vi "Configure Math.vi"(0 "VISA resource name":refnum<visa-resource-name>, 1 "Operation (0:None)":T1(ring), 2 "Internal Math Buffer Storage (T: Enabled)":bool=TRUE, 5 "Null Offset (0.00)":dbl format="%_3f", 7 "dB Reference Point (0.00 dB)":dbl format="%.2f", 9 "dBm Resistance (600 Ohms)":i32(ring)=600 items=["50"=50, "75"=75, "93"=93, "110"=110, "124"=124, "125"=125, "135"=135, "150"=150, "250"=250, "300"=300, "500"=500, "600"=600, "800"=800, "900"=900, "1000"=1000, "1200"=1200, "8000"=8000], 11 "error in (no error)":errorcluster, 12 "Upper Limit (0.00)":dbl format="%.2f", 13 "Lower Limit (0.00)":dbl format="%.2f") -> (4 "VISA resource name out":refnum<visa-resource-name>, 15 "error out":errorcluster)   [LabVIEW 2013, in "Agilent 34401.lvlib"]
doc: "Configures the math functions available on the instrument."
uses:
  <instrlib>/Agilent 34401/Agilent 34401.lvlib
panel:
  # "Limit"
  # "Null Function"
  # "DB Measurements"
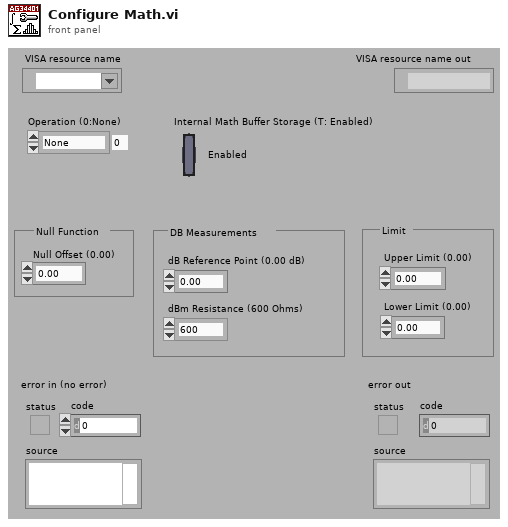
[diagram p1: front panel]
types:
  T1 = enum16{"None", "Min/Max", "Null", "dB", "dBm", "Limit"}
  T2 = typedef "Agilent 34401.lvlib/Extended User Data.ctl" = cluster{"Trigger Source":u16, "Math Storage":u16, "Agilent Model":i32}
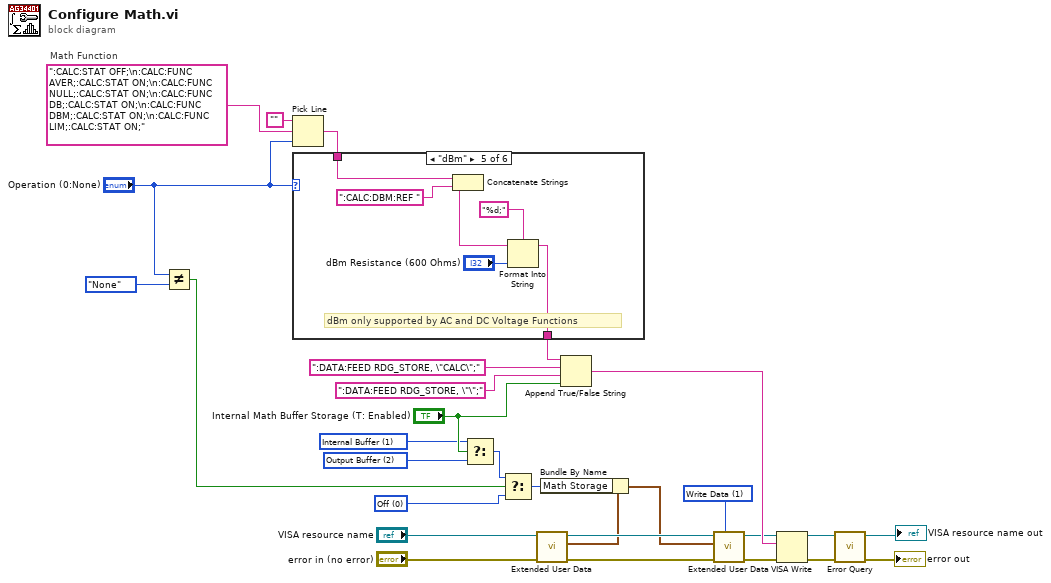
[diagram p0: block diagram]
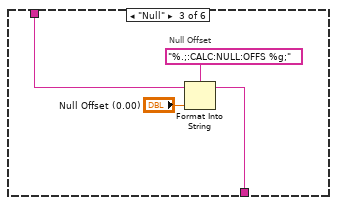
[diagram p4: hidden frame]
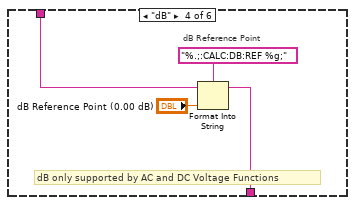
[diagram p5: hidden frame]
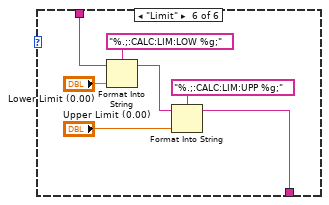
[diagram p6: hidden frame]
diagram:
  w1 = u16 1 items=["Read Data", "Write Data", "Dispose of Data"] ("Action")
  w6 = u16 0 items=["Off", "Internal Buffer", "Output Buffer"] ("Math Storage")
  w7 = u16 2 items=["Off", "Internal Buffer", "Output Buffer"] ("Math Storage")
  w8 = u16 1 items=["Off", "Internal Buffer", "Output Buffer"] ("Math Storage")
  # "Math Function"
  n1 = Not Equal?(x="Operation (0:None)", y=T1."None") -> (x != y?=w5:bool)
  n2 = Pick Line(string ("")="" ("Empty String Constant"), multi-line string=":CALC:STAT OFF;\n:CALC:FUNC AVER;:CALC:STAT ON;\n:CALC:FUNC NULL;:CALC:STAT ON;\n:CALC:FUNC DB;:CALC:STAT ON;\n:CALC:FUNC DBM;:CALC:STAT ON;\n:CALC:FUNC LIM;:CALC:STAT ON;", line index="Operation (0:None)") -> (output string=w28:string)
  n3 = case shown="\"dBm\"" "Operation (0:None)" {
    tunnel: w28 -> [w30 w31 w35 w39 w45 w52]
    tunnel: [w30 w31 w34 w37 w40 w46] -> w20
    frame "None", Default {
    }
    frame "Min/Max" {
    }
    frame "Null" {
      # "Null Offset"
      n4 = Format Into String(format string="%.;:CALC:NULL:OFFS %g;", initial string=w35, "Null Offset (0.00)") -> (resulting string=w34:string)  [unwired: 1 in, 1 out]
    }
    frame "dB" {
      # "dB only supported by AC and DC Voltage Functions"
      # "dB Reference Point"
      n5 = Format Into String(format string="%.;:CALC:DB:REF %g;", initial string=w39, "dB Reference Point (0.00 dB)") -> (resulting string=w37:string)  [unwired: 1 in, 1 out]
    }
    frame "dBm" {
      # "dBm only supported by AC and DC Voltage Functions"
      n6 = Concatenate Strings(w45, ":CALC:DBM:REF ") -> (w43:string)
      n7 = Format Into String(format string="%d;", initial string=w43, "dBm Resistance (600 Ohms)") -> (resulting string=w40:string)  [unwired: 1 in, 1 out]
    }
    frame "Limit" {
      n8 = Format Into String(format string="%.;:CALC:LIM:LOW %g;", initial string=w52, "Lower Limit (0.00)") -> (resulting string=w47:string)  [unwired: 1 in, 1 out]
      n9 = Format Into String(format string="%.;:CALC:LIM:UPP %g;", initial string=w47, "Upper Limit (0.00)") -> (resulting string=w46:string)  [unwired: 1 in, 1 out]
    }
  }
  n10 = Select(t=w8, s="Internal Math Buffer Storage (T: Enabled)", f=w7) -> (s? t:f=w4:u16)
  n11 = Select(t=w4, s=w5, f=w6) -> (s? t:f=w3:u16)
  n12 = call <instrlib>:"Extended User Data.vi"("Error In (no error)"="error in (no error)", "VISA resource name in"="VISA resource name") -> ("Error Out"=w12:errorcluster, "User Data Out"=w10:T2, "VISA resource name out"=w11:refnum<visa-resource-name>)  [unwired: 7 in]
  n13 = Bundle By Name(cluster=w10, "Math Storage"=w3) -> (w2:T2)
  n14 = Append True/False String(1:"Internal Math Buffer Storage (T: Enabled)", 2:":DATA:FEED RDG_STORE, \"\";" ("true string"), 3:":DATA:FEED RDG_STORE, \"CALC\";" ("true string"), 4:w20) -> (0:w19:string)
  n15 = call <instrlib>:"Extended User Data.vi"("Action"=w1, "Error In (no error)"=w12, "User Data In"=w2, "VISA resource name in"=w11) -> ("Error Out"=w17:errorcluster, "VISA resource name out"=w18:refnum<visa-resource-name>)  [unwired: 5 in, 1 out]
  n16 = VISA Write(VISA resource name=w18, write buffer=w19, error in (no error)=w17) -> (VISA resource name out=w25:refnum<visa-resource-name>, error out=w26:errorcluster)  [unwired: 1 out]
  n17 = call <instrlib>:"Error Query.vi"("error in (no error)"=w26, "VISA resource name"=w25) -> ("error out"=→"error out":errorcluster, "VISA resource name out"=→"VISA resource name out":refnum<visa-resource-name>)  [unwired: 6 in, 2 out]
